vi "VISA config.vi"() -> ()   [LabVIEW 2012]
uses:
  <vilib>/Instr/_visa.llb/VISA Find Search Mode.ctl
  <vilib>/Instr/_visa.llb/VISA Configure Serial Port (Instr).vi
panel:
  in  "wait (ms)":u32=7000
  in  "INIT* mode":bool=TRUE
  in  "data3":string="C0"
  in  "data2":string="06"
  in  "data1":string="05"
  in  "cmd":string="FD"
  in  "add":u8 format="%0.0f"
  out "Checksum ok?":bool
  out "chk":u8 format="%x"
  out "term":string="\r"
  out "Output to device":string="%00FD0506C0\r"
  in  "bytes to read":u32=64
  in  "flow control (0:none)":u16(ring) items=["None", "XON/XOFF", "RTS/CTS", "XON/XOFF & RTS/CTS", "DTR/DSR", "XON/XOFF & DTR/DSR"]
  in  "stop bits":u16(ring)=10 items=["1.0"=10, "1.5"=15, "2.0"=20]
  in  "parity":enum16{"None", "Odd", "Even", "Mark", "Space"}(ring)
  in  "data bits":u16=8 min=5 max=8 step=1
  in  "baud rate (bps)":u32=9600
  in  "timeout (ms)":u32=1000
  in  "enable termination char":bool=TRUE
  in  "termination char":u8=13 format="%.0x"
  out "bytes returned":u32=4
  out "Error":errorcluster
  out "Response from device":string="!FD\r"
  out "bytes written":u32=12
  in  "del":string="%"
  in  "VISA resource name":refnum<visa-resource-name>="COM3"
  out "Port list":string[](array[string])=["COM1", "COM3"]
  # "(hex)"
  # "(hex)"
  # "(dec)"
  # "(hex)"
  # "(hex)"
  # "(hex)"
  # "(str)"
  # "(str)"
  # "(no checksum in INIT* mode)"
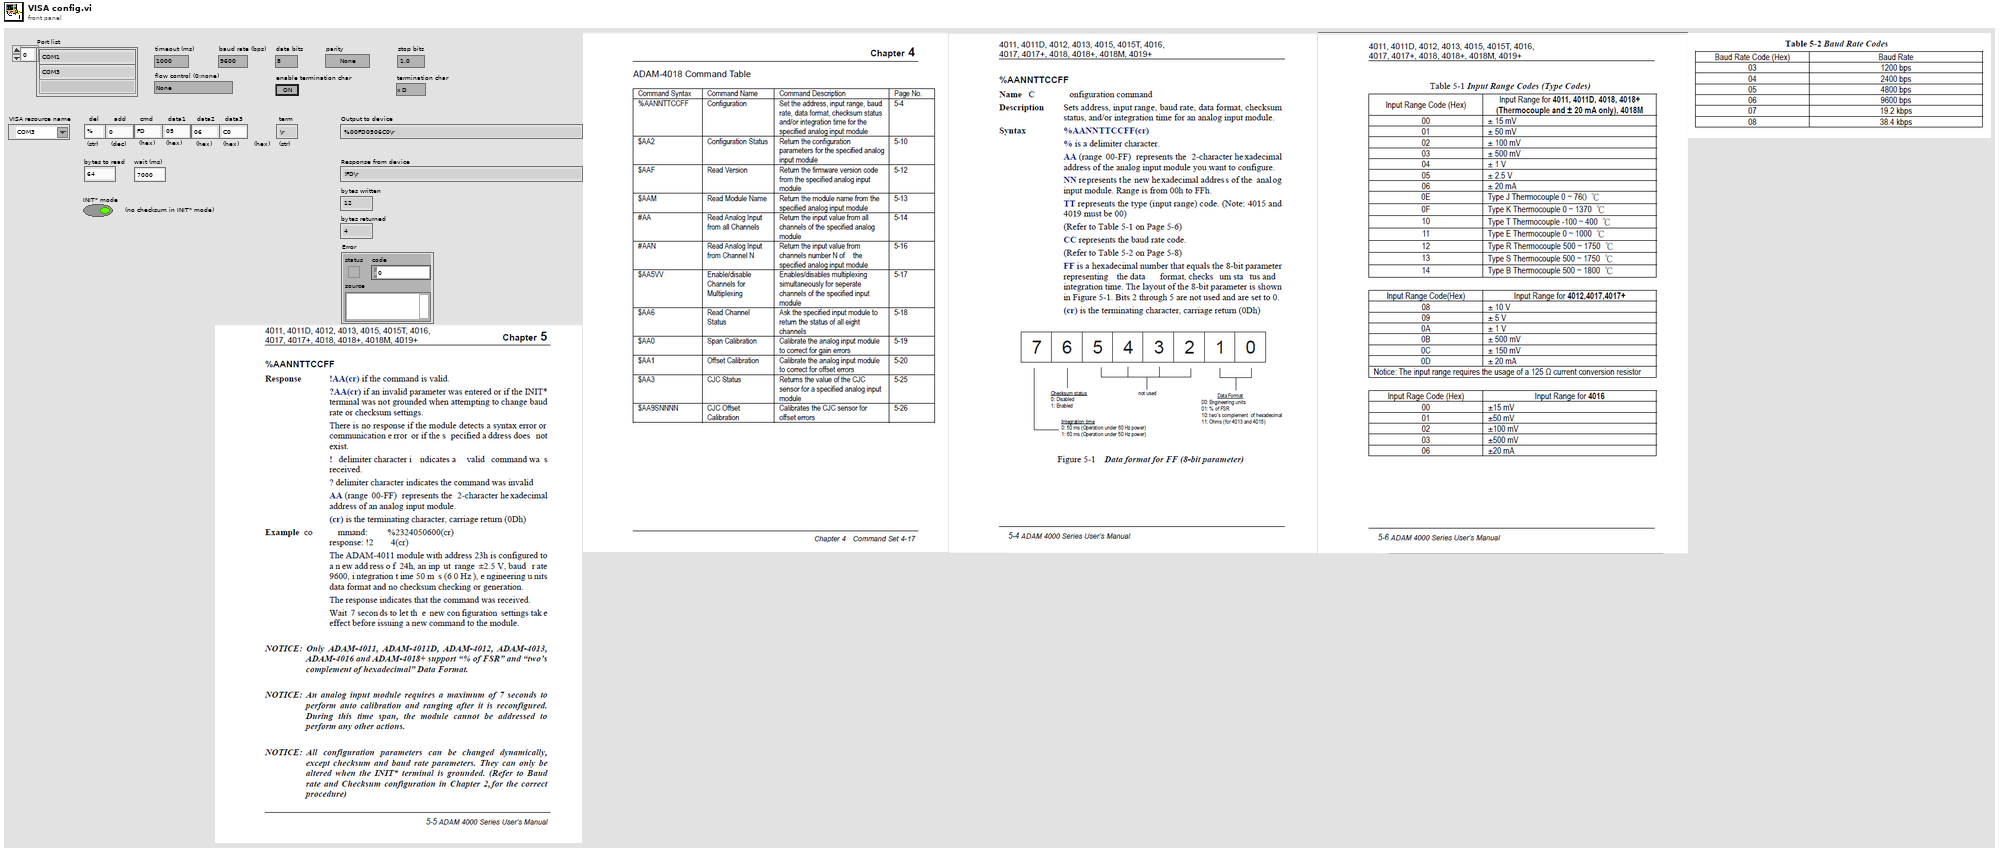
[diagram p1: front panel]
types:
  T1 = typedef "VISA Find Search Mode.ctl" = u32
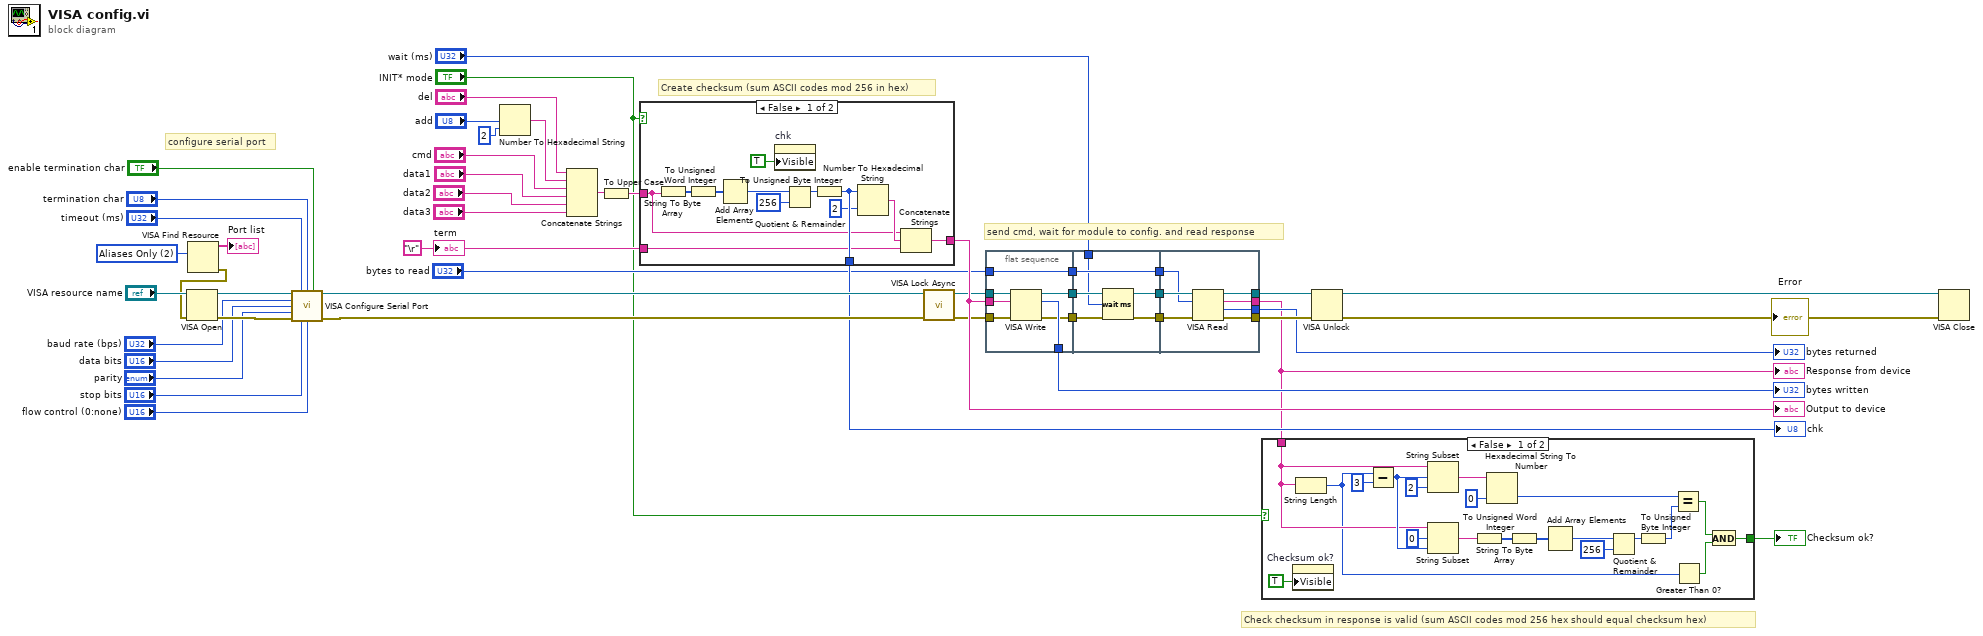
[diagram p0: block diagram]
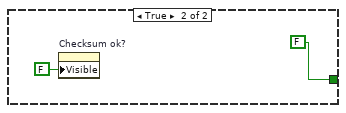
[diagram p2: hidden frame]
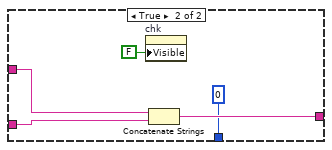
[diagram p3: hidden frame]
diagram:
  w25 = "\r"
  w47 = T1 2 items=["Canonical Names Only"=0, "Aliases Only"=2, "Include Matching Aliases"=3, "Include All Aliases"=4] ("Search Mode")
  # "configure serial port"
  # "Check checksum in response is valid (sum ASCII codes mod 256 hex should equal checksum hex)"
  # "send cmd, wait for module to config. and read response"
  # "Create checksum (sum ASCII codes mod 256 in hex)"
  n1 = VISA Find Resource(10:w47) -> (0:w45:errorcluster, 3:→"Port list":string[])  [unwired: 2 in, 1 out]
  n2 = VISA Open(error in (no error)=w45, VISA resource name="VISA resource name") -> (VISA resource name=w44:refnum<visa-resource-name>, error out=w43:errorcluster)  [unwired: 3 in]
  n3 = call-poly "VISA Configure Serial Port"("VISA resource name"=w44, "timeout (10sec)"="timeout (ms)", "termination char\n(0xA = '\\n' = LF)"="termination char", "Enable Termination\nChar (T)"="enable termination char", "baud rate (9600)"="baud rate (bps)", "data bits (8)"="data bits", "parity (0:none)"="parity", "error in (no error)"=w43, "stop bits (10: 1 bit)"="stop bits", "flow control (0:none)"="flow control (0:none)") -> ("VISA resource name out"=w34:refnum<visa-resource-name>, "error out"=w33:errorcluster)  [unwired: 4 in]
  n4 = Number To Hexadecimal String(1:i16 2 ("width (-)"), 2:"add") -> (0:w22:string)
  n5 = Concatenate Strings("del", w22, "cmd", "data1", "data2", "data3") -> (w15:string)
  n6 = To Upper Case(1:w15) -> (0:w14:string)
  n7 = case shown="False" "INIT* mode" {
    tunnel: [w60 w64] -> w29
    tunnel: [w59 u8 0] -> w28
    tunnel: w25 -> [w58 w65]
    tunnel: w14 -> [w50 w63]
    frame False {
      n8 = String To Byte Array(string=w50) -> (unsigned byte array=w53:u8[])
      n9 = To Unsigned Word Integer(number=w53) -> (unsigned 16bit integer=w52:u16[])
      n10 = Add Array Elements(numeric array=w52) -> (sum=w51:u16)
      n11 = property on="chk" class="DigNum (strict)"("Visible"=TRUE) -> ()  [unwired: 2 in, 2 out]
      n12 = Quotient & Remainder(x=w51, y=u16 256) -> (x-y*floor(x/y)=w56:u16)  [unwired: 1 out]
      n13 = To Unsigned Byte Integer(number=w56) -> (unsigned 8bit integer=w59:u8)
      n14 = Number To Hexadecimal String(1:i16 2 ("width (-)"), 2:w59) -> (0:w54:string)
      n15 = Concatenate Strings(w50, w54, w58) -> (w60:string)
    }
    frame True {
      n16 = property on="chk" class="DigNum (strict)"("Visible"=FALSE) -> ()  [unwired: 2 in, 2 out]
      n17 = Concatenate Strings(w63, w65) -> (w64:string)
    }
  }
  "Output to device" <- w29
  "chk" <- w28
  n18 = call <vilib>:"VISA Lock Async.vi"("error in (no error)"=w33, "VISA resource name"=w34) -> ("error out"=w19:errorcluster, "VISA resource name out"=w18:refnum<visa-resource-name>)  [unwired: 7 in, 1 out]
  n19 = flat-sequence {
    tunnel: [w72] -> w30
    tunnel: w29 -> [w71]
    tunnel: w19 -> [w70]
    tunnel: w18 -> [w69]
    tunnel: [w68] -> w13
    tunnel: [w67] -> w11
    tunnel: "bytes to read" -> [w66]
    tunnel: [w66] -> w7
    tunnel: w13 -> [w76]
    tunnel: [w76] -> w12
    tunnel: w11 -> [w75]
    tunnel: [w75] -> w10
    tunnel: [w74] -> w8
    tunnel: w7 -> [w74]
    tunnel: "wait (ms)" -> [w73]
    tunnel: w12 -> [w81]
    tunnel: w10 -> [w80]
    tunnel: w8 -> [w77]
    tunnel: [w83] -> w6
    tunnel: [w82] -> w5
    tunnel: [w79] -> w4
    tunnel: [w78] -> w3
    frame #0 {
      n20 = VISA Write(VISA resource name=w69, write buffer=w71, error in (no error)=w70) -> (VISA resource name out=w68:refnum<visa-resource-name>, return count=w72:u32, error out=w67:errorcluster)
    }
    frame #1 {
      n21 = Wait (ms)(milliseconds to wait=w73) -> ()  [unwired: 1 out]
    }
    frame #2 {
      n22 = VISA Read(VISA resource name=w81, byte count=w77, error in (no error)=w80) -> (VISA resource name out=w83:refnum<visa-resource-name>, read buffer=w78:string, return count=w79:u32, error out=w82:errorcluster)
    }
  }
  n23 = case shown="False" "INIT* mode" {
    tunnel: [w84 FALSE] -> w27
    tunnel: w3 -> [w89 _]
    frame False {
      n24 = property on="Checksum ok?" class="Bool (strict)"("Visible"=TRUE) -> ()  [unwired: 2 in, 2 out]
      n25 = String Length(string=w89) -> (length=w87:i32)
      n26 = Subtract(x=w87, y=3) -> (x-y=w100:i32)
      n27 = String Subset(string=w89, offset (0)=w100, length (rest)=2 ("length (rest)")) -> (substring=w92:string)
      n28 = String Subset(string=w89, offset (0)=0, length (rest)=w100) -> (substring=w99:string)
      n29 = String To Byte Array(string=w99) -> (unsigned byte array=w98:u8[])
      n30 = Hexadecimal String To Number(string=w92, default (0uL)=u8 0 ("default (0 U32)")) -> (number=w90:u8)  [unwired: 1 in, 1 out]
      n31 = To Unsigned Word Integer(number=w98) -> (unsigned 16bit integer=w93:u16[])
      n32 = Add Array Elements(numeric array=w93) -> (sum=w94:u16)
      n33 = Quotient & Remainder(x=w94, y=u16 256) -> (x-y*floor(x/y)=w97:u16)  [unwired: 1 out]
      n34 = To Unsigned Byte Integer(number=w97) -> (unsigned 8bit integer=w95:u8)
      n35 = Equal?(x=w90, y=w95) -> (x = y?=w86:bool)
      n36 = Greater Than 0?(x=w87) -> (x > 0?=w85:bool)
      n37 = And(x=w86, y=w85) -> (x .and. y?=w84:bool)
    }
    frame True {
      n38 = property on="Checksum ok?" class="Bool (strict)"("Visible"=FALSE) -> ()  [unwired: 2 in, 2 out]
    }
  }
  "Checksum ok?" <- w27
  n39 = VISA Unlock(8:w5, 11:w6) -> (0:w31:errorcluster, 3:w32:refnum<visa-resource-name>)
  "Error" <- w31
  n40 = VISA Close(VISA resource name=w32, error in (no error)=w31) -> ()  [unwired: 1 out]
  "bytes written" <- w30
  "Response from device" <- w3
  "bytes returned" <- w4
  "term" <- w25
